vi "ADC_GRAPH_REQ.vi"(0 "Gain 2":dbl, 1 "Numeric":i32, 3 "ch":u8, 4 "Rsense 2":dbl, 5 "Buffer":i32, 7 "aDATA":u8[](array[numeric]), 8 "Array":T1(array[cluster]), 9 "Curr 1":u16(ring) items=["Vin", "Vout", "Curren", "Temp"], 12 "index Ch1":i32, 13 "index Ch2":i32, 14 "ch1_old":dbl, 15 "ch2_old":dbl, 16 "Ring":u16(ring) items=["None", "Status", "ADC", "Status&ADC", "Temperature", "Graph", "Params"], 17 "Curr 2":u16(ring) caption="Ch2" items=["Vin", "Vout", "Curren", "Temp"]) -> (18 "ADC UnitT3":dbl, 19 "ADC UnitT4":dbl, 20 "ADC Units 1":dbl, 21 "Arr Out":T1(array[cluster]), 22 "ADC UnitT1":dbl, 23 "ADC UnitT2":dbl, 24 "ch1_oldout":dbl, 25 "num out":i32, 27 "ch2_oldout":dbl)   [LabVIEW 2017]
panel:
  out "ADC Units 2":dbl
  out "ADC Unit2":dbl
  out "ADC Units":dbl
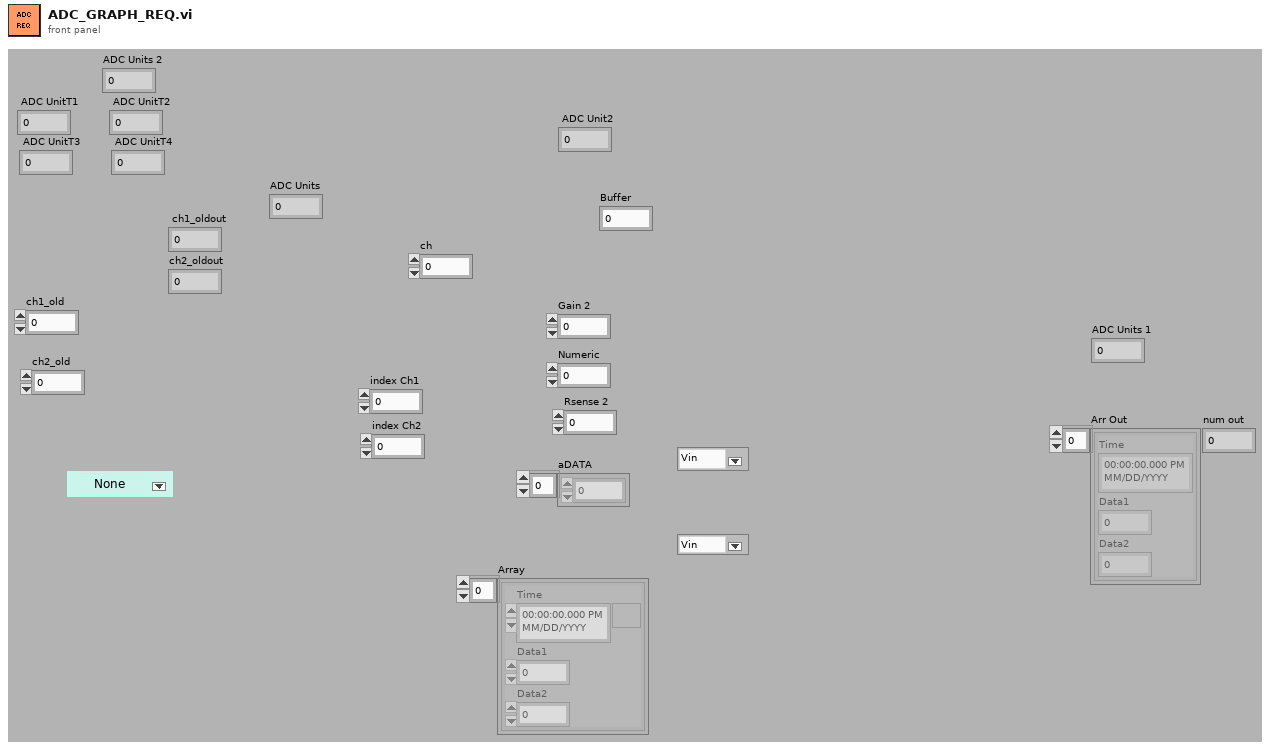
[diagram p1: front panel]
types:
  T1 = cluster{"Time":timestamp, "Data1":dbl, "Data2":dbl}[]
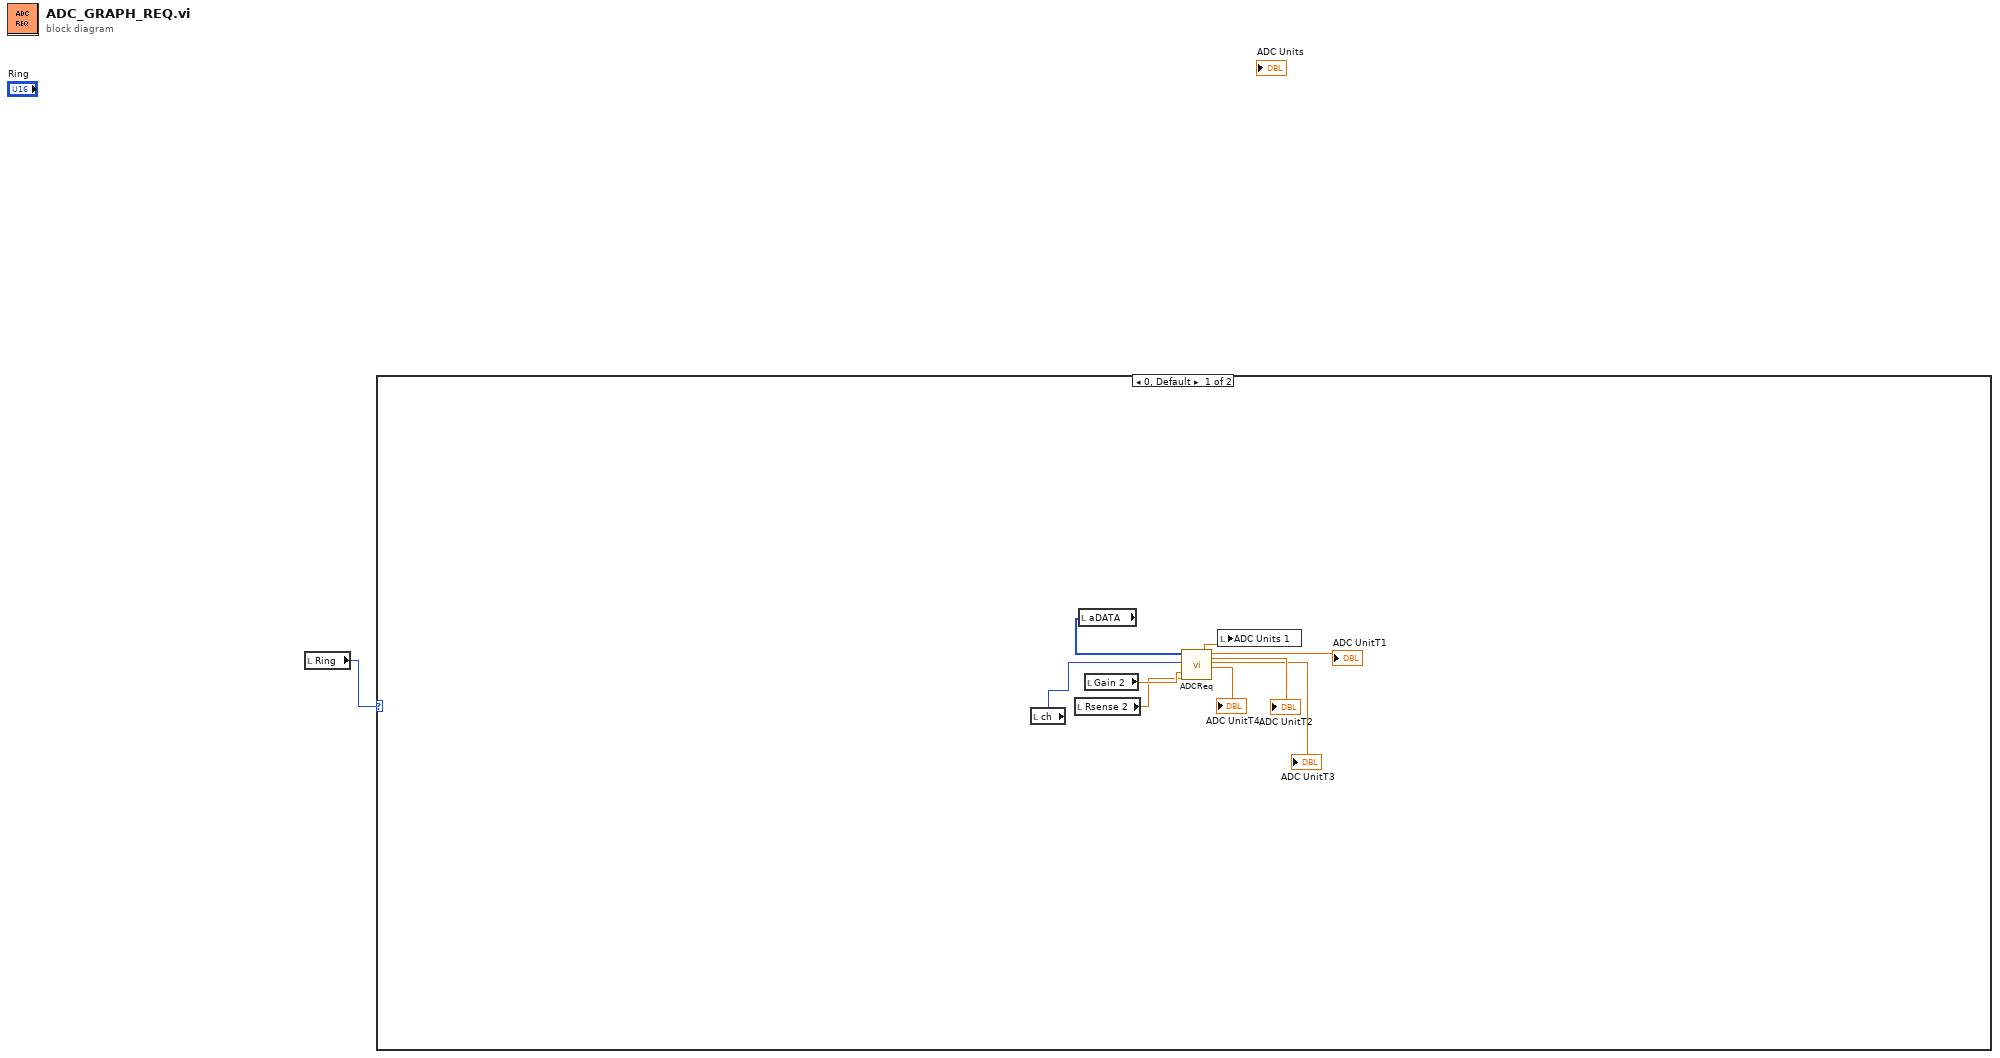
[diagram p0: block diagram]
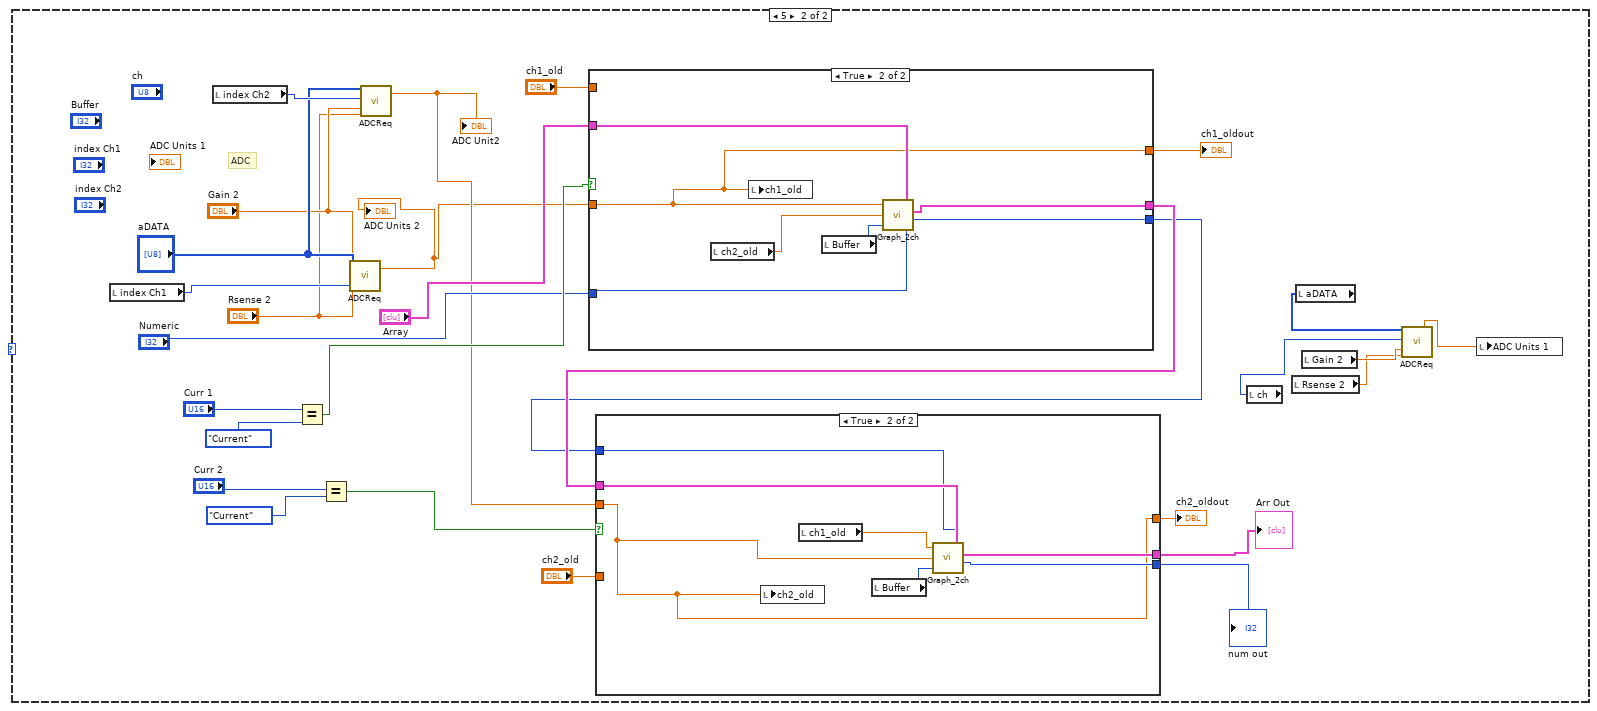
[diagram p2: hidden frame]
diagram:
  n1 = local read "Ring"() -> (w1:u16)
  n2 = case shown="0, Default" w1 {
    frame 0, Default {
      n3 = local read "ch"() -> (w6:u8)
      n4 = local read "Rsense 2"() -> (w9:dbl)
      n5 = local read "aDATA"() -> (w8:u8[])
      n6 = local read "Gain 2"() -> (w10:dbl)
      n7 = call "ADCReq.vi"("aDATA"=w8, "ch"=w6, "Gain"=w10, "Rsense"=w9) -> ("ADC Unit"=w7:dbl, "ADC UnitT1"=→"ADC UnitT1":dbl, "ADC UnitT2"=→"ADC UnitT2":dbl, "ADC UnitT3"=→"ADC UnitT3":dbl, "ADC UnitT4"=→"ADC UnitT4":dbl)  [unwired: 11 in]
      n8 = local write "ADC Units 1"(w7) -> ()
    }
    frame 5 {
      # "ADC"
      n9 = local read "index Ch1"() -> (w34:i32)
      n10 = local read "index Ch2"() -> (w33:i32)
      n11 = Equal?(x="Curr 1", y=enum16{"Vin", "Vout", "Current", "Temp"}."Current" ("Ch1 2")) -> (x = y?=w24:bool)
      n12 = Equal?(x="Curr 2", y=enum16{"Vin", "Vout", "Current", "Temp"}."Current" ("Ch1 2")) -> (x = y?=w23:bool)
      n13 = call "ADCReq.vi"("aDATA"="aDATA", "ch"=w34, "Gain"="Gain 2", "Rsense"="Rsense 2") -> ("ADC Unit"=w12:dbl)  [unwired: 11 in, 4 out]
      "ADC Units 2" <- w12
      n14 = call "ADCReq.vi"("aDATA"="aDATA", "ch"=w33, "Gain"="Gain 2", "Rsense"="Rsense 2") -> ("ADC Unit"=w17:dbl)  [unwired: 11 in, 4 out]
      "ADC Unit2" <- w17
      n15 = case shown="True" w24 {
        tunnel: [w40 w47] -> w29
        tunnel: [w39 w46] -> w27
        tunnel: "Array" -> [w40 w45]
        tunnel: w12 -> [_ w42]
        tunnel: "Numeric" -> [w39 w44]
        tunnel: [w41 w42] -> w21
        tunnel: "ch1_old" -> [w41 _]
        frame False {
        }
        frame True {
          n16 = local read "ch2_old"() -> (w43:dbl)
          n17 = local write "ch1_old"(w42) -> ()
          n18 = local read "Buffer"() -> (w48:i32)
          n19 = call "Graph_2ch.vi"("Buff Len"=w48, "ch2"=w43, "ch1"=w42, "num in"=w44, "ArrayIn"=w45) -> ("num out"=w46:i32, "Arr Out"=w47:T1)
        }
      }
      "ch1_oldout" <- w21
      n20 = case shown="True" w23 {
        tunnel: w29 -> [w51 w57]
        tunnel: [w51 w56] -> w28
        tunnel: w27 -> [w50 w55]
        tunnel: [w50 w54] -> w26
        tunnel: w17 -> [_ w52]
        tunnel: [w49 w52] -> w20
        tunnel: "ch2_old" -> [w49 _]
        frame False {
        }
        frame True {
          n21 = local write "ch2_old"(w52) -> ()
          n22 = local read "ch1_old"() -> (w53:dbl)
          n23 = local read "Buffer"() -> (w58:i32)
          n24 = call "Graph_2ch.vi"("Buff Len"=w58, "ch2"=w52, "ch1"=w53, "num in"=w55, "ArrayIn"=w57) -> ("num out"=w54:i32, "Arr Out"=w56:T1)
        }
      }
      "Arr Out" <- w28
      "num out" <- w26
      "ch2_oldout" <- w20
      n25 = local read "ch"() -> (w11:u8)
      n26 = local read "Rsense 2"() -> (w15:dbl)
      n27 = local read "aDATA"() -> (w14:u8[])
      n28 = local read "Gain 2"() -> (w16:dbl)
      n29 = call "ADCReq.vi"("aDATA"=w14, "ch"=w11, "Gain"=w16, "Rsense"=w15) -> ("ADC Unit"=w13:dbl)  [unwired: 11 in, 4 out]
      n30 = local write "ADC Units 1"(w13) -> ()
    }
  }
